vi "PreCalc Frame Durations.vi"(8 "error in (no error)":errorcluster, 10 "Baud Rate":u64=125000, 11 "CAN Bus Class In":refnum<class "CANBus_Load_Calculator.lvclass">) -> (0 "error out":errorcluster, 3 "CAN Bus Class Out":refnum<class "CANBus_Load_Calculator.lvclass">)   [LabVIEW 2019, in "XNET-Bus-Load-Calculator.lvlib" / "CANBus_Load_Calculator.lvclass"]
uses:
  CANBus_Load_Calculator.lvclass
panel:
  in  "FD Baud Rate":u64=1000000
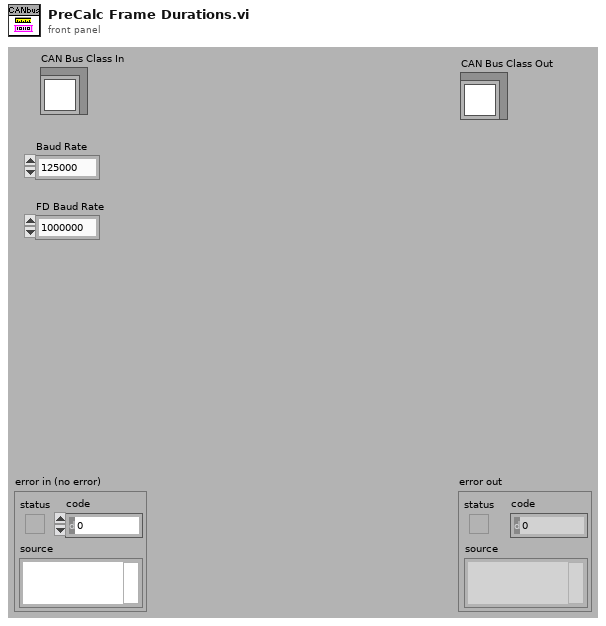
[diagram p1: front panel]
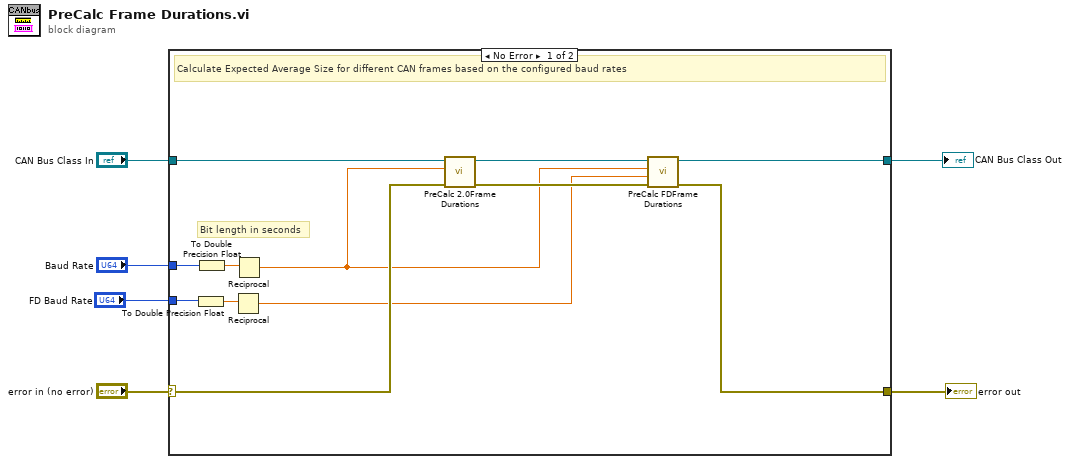
[diagram p0: block diagram]
diagram:
  n1 = case shown="No Error" "error in (no error)" {
    selector: "error in (no error)" -> [w13 w20]
    tunnel: [w9 w20] -> w5
    tunnel: "Baud Rate" -> [w18 _]
    tunnel: "CAN Bus Class In" -> [w16 w19]
    tunnel: [w11 w19] -> w2
    tunnel: "FD Baud Rate" -> [w14 _]
    frame No Error {
      # "Bit length in seconds"
      # "Calculate Expected Average Size for different CAN frames based on the configured baud rates"
      n2 = To Double Precision Float(number=w14) -> (double precision float=w15:dbl)
      n3 = To Double Precision Float(number=w18) -> (double precision float=w17:dbl)
      n4 = Reciprocal(x=w15) -> (1/x=w7:dbl)
      n5 = Reciprocal(x=w17) -> (1/x=w8:dbl)
      n6 = call "PreCalc 2.0Frame Durations.vi"("error in (no error)"=w13, "Bit Time (seconds)"=w8, "CANBus_Load_Calculator in"=w16) -> ("error out"=w10:errorcluster, "CANBus_Load_Calculator out"=w12:refnum<class "CANBus_Load_Calculator.lvclass">)  [unwired: 7 in]
      n7 = call "PreCalc FDFrame Durations.vi"("error in (no error)"=w10, "Bit Time FD (seconds)"=w7, "Bit Time (seconds)"=w8, "CANBus_Load_Calculator in"=w12) -> ("error out"=w9:errorcluster, "CANBus_Load_Calculator out"=w11:refnum<class "CANBus_Load_Calculator.lvclass">)  [unwired: 6 in]
    }
    frame Error {
    }
  }
  "CAN Bus Class Out" <- w2
  "error out" <- w5
